vi "NewData.vi"(2 "Ext":string=".txt", 3 "Prefix":string, 4 "data location":path=path "G:/Data") -> (0 "data file name":string, 1 "data file refnum":refnum<file>)   [LabVIEW 2014]
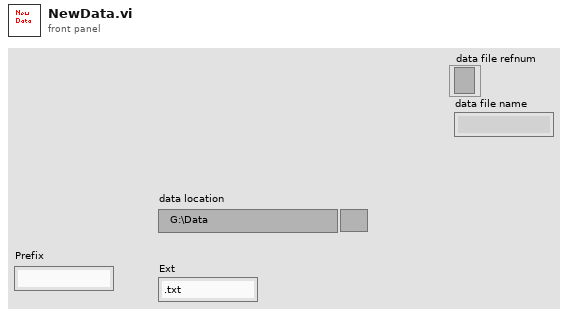
[diagram p1: front panel]
types:
  T1 = enum16{"open", "replace", "create", "open or create", "replace or create", "replace or create with confirmation"}
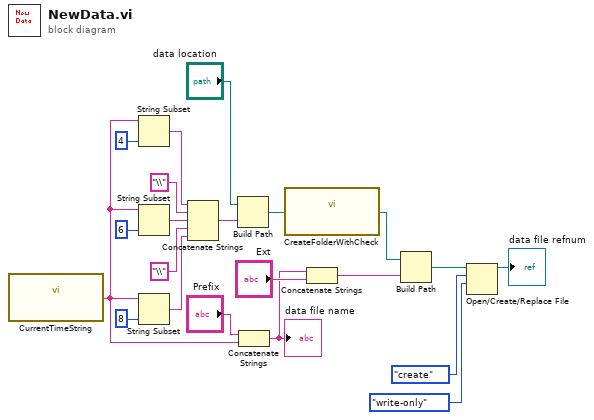
[diagram p0: block diagram]
diagram:
  n1 = call "CurrentTimeString.vi"() -> ("date/time string"=w10:string)
  n2 = String Subset(string=w10, length (rest)=4 ("length (rest)")) -> (substring=w18:string)  [unwired: 1 in]
  n3 = String Subset(string=w10, length (rest)=6 ("length (rest)")) -> (substring=w16:string)  [unwired: 1 in]
  n4 = String Subset(string=w10, length (rest)=8 ("length (rest)")) -> (substring=w14:string)  [unwired: 1 in]
  n5 = Concatenate Strings(w18, "\\" ("string"), w16, "\\" ("string"), w14) -> (w13:string)
  n6 = Build Path(base path="data location", name or relative path=w13) -> (appended path=w9:path)
  n7 = Concatenate Strings("Prefix", w10) -> (w4:string)
  "data file name" <- w4
  n8 = call "CreateFolderWithCheck.vi"("path"=w9) -> ("created path"=w2:path)
  n9 = Concatenate Strings(w4, "Ext") -> (w3:string)
  n10 = Build Path(base path=w2, name or relative path=w3) -> (appended path=w1:path)
  n11 = Open/Create/Replace File(file path (use dialog)=w1, operation (0:open)=T1."create", access (0:read/write)=enum16{"read/write", "read-only", "write-only"}."write-only") -> (refnum out=→"data file refnum":refnum<file>)  [unwired: 3 in, 2 out]
